vi "Transmit Data.vi"(8 "error in (no error)":errorcluster, 10 "Data":i32[](array[numeric]), 11 "RP Transceiver in":refnum<class "RP Transceiver.lvclass">) -> (0 "error out":errorcluster, 3 "RP Transceiver out":refnum<class "RP Transceiver.lvclass">)   [LabVIEW 2015, in "RP Transceiver.lvclass"]
uses:
  RP Transceiver.lvclass
  RP Transceiver.lvclass/RP Transceiver.ctl
  RP Communicator/RP Communicator.lvclass
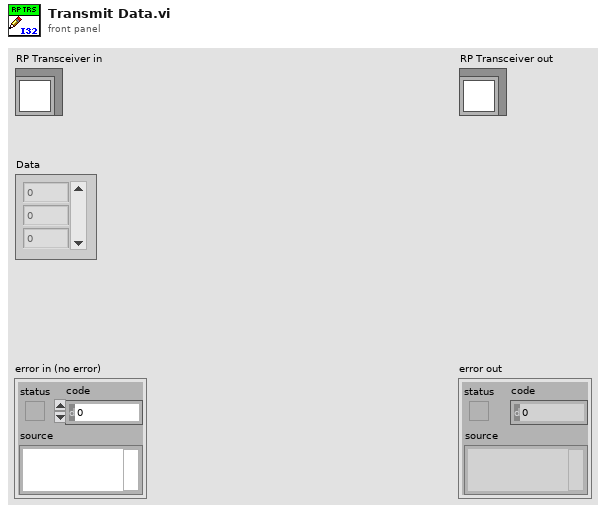
[diagram p1: front panel]
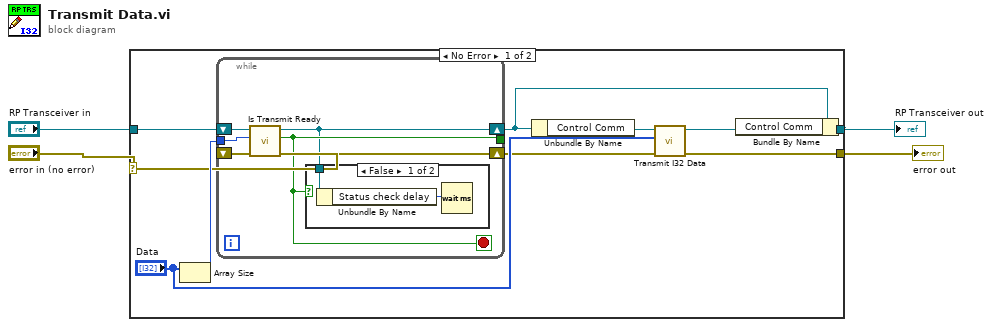
[diagram p0: block diagram]
diagram:
  n1 = case shown="No Error" "error in (no error)" {
    selector: "error in (no error)" -> [w6 w24]
    tunnel: [w10 w24] -> w3
    tunnel: [w12 w23] -> w1
    tunnel: "RP Transceiver in" -> [w9 w23]
    frame No Error {
      n2 = Array Size(array="Data") -> (size(s)=w7:i32)
      n3 = while {
        shift-right: [w18] -> w5
        shift-left: w6 -> [w19]
        shift-right: [w15] -> w8
        shift-left: w9 -> [w20]
        tunnel: [w17] -> _
        tunnel: w7 -> [w16]
        stop <- w17 stop-if-true
        n4 = call-dynamic "Is Transmit Ready.vi"("error in (no error)"=w19, "Samples to transmit"=w16, "RP Lockin in"=w20) -> ("error out"=w18:errorcluster, "Transmit Ready"=w17:bool, "RP Lockin out"=w15:refnum<class "RP Transceiver.lvclass">)  [unwired: 6 in]
        n5 = case shown="False" w17 {
          tunnel: w15 -> [w22 _]
          frame False {
            n6 = Unbundle By Name(w22) -> ("Status check delay"=w21:u32)
            n7 = Wait (ms)(milliseconds to wait=w21) -> ()  [unwired: 1 out]
          }
          frame True {
          }
        }
      }
      n8 = Unbundle By Name(w8) -> ("Control Comm"=w14:refnum<class "RP Communicator.lvclass">)
      n9 = call-dynamic "Transmit I32 Data.vi"("error in (no error)"=w5, "Data"="Data", "RP Communicator in"=w14) -> ("error out"=w10:errorcluster, "RP Communicator out"=w13:refnum<class "RP Communicator.lvclass">)  [unwired: 7 in]
      n10 = Bundle By Name(cluster=w8, "Control Comm"=w13) -> (w12:refnum<class "RP Transceiver.lvclass">)
    }
    frame Error {
    }
  }
  "error out" <- w3
  "RP Transceiver out" <- w1
